vi "Robotiq Control.vi"() -> ()   [LabVIEW 2013]
uses:
  Common/controls/Robotiq Mode.ctl
  Common/classes/MF3/MF3.lvclass
  robotiq_labview/Class/Robotiq.lvclass
  Common/controls/Robotiq Positions.ctl
  labview_ros/std_msgs/Bool.ctl
  <vilib>/Platform/TimedLoop/XDataNode/timing_clust.ctl
  <vilib>/Platform/TimedLoop/XDataNode/nitl_modes.ctl
  <vilib>/Platform/TimedLoop/XDataNode/wakeup.ctl
  labview_ros/takktile_msgs/RobotiqTouch.ctl
  robotiq_labview/Controls/Gripper Command.ctl
  robotiq_labview/Controls/Finger Command.ctl
  <vilib>/Analysis/baseanly.llb/Unit Vector (DBL).vi
  <vilib>/Analysis/1siggen.llb/Riffle Array (I32) (obs 2012).vi
  <userlib>/_matio/level5/Public/Write/Append Data Element.llb/Append Data Element (1D Array of Double).vi
  <userlib>/_matio/level5/Public/Write/Append Data Element.llb/Append Data Element (2D Array of Double).vi
  <vilib>/Platform/TimedLoop/XDataNode/XDataNode.xnode
  <userlib>/_matio/level5.lvlib
  <vilib>/Platform/TimedLoop/XDataNode/XDNodeRunTimeDep.lvlib
  <vilib>/Analysis/NI_AALBase.lvlib
panel:
  in  "Gains":dbl[](array[numeric])=[3.0, 3.0, 3.0, 0.0, 0.0, 0.0, 0.0, 0.0, 0.0]
  out "Finger 3":T1
  out "Finger 2":T1
  out "Finger 1":T1
  out "Takktile Sender":errorcluster
  in  "Takktile":T2={"IP"="192.168.0.10", "Read Port"=5051, "Write Port"=5052}
  in  "Zero Takktile":bool
  out "Target Grasp":cluster{"Mode":T3, "Number":i32}={"Mode"=enum."Basic", "Number"=0}
  in  "OK Button":bool
  out "dp":T4(graph)
  out "velocities":T4(graph)
  out "area":dbl(graph)
  out "Requested?":bool caption="Time has Elapsed"
  in  "Transition time (s)":dbl=0.5 caption="Time Target (s)"
  out "Robotiq Mode":T3
  out "Takktile Rate":dbl
  in  "MasterFinger":T5={"PID Gains"={"Proportional Gain"=20, "Integral Gain"=5, "Derivative Gain"=0}, "Current limit"=0.0}
  in  "Data Logging":cluster{"Path":path, "Save":bool}={"Path"=path "c:/ni-rt/testing/grasping.mat", "Save"=TRUE}
  out "Logging Status":errorcluster
  out "Takktile Receiver":errorcluster
  in  "Robotiq Hand":cluster{"IP":string, "Port":u16, "Move":bool}={"IP"="192.168.0.8", "Port"=502, "Move"=FALSE}
  out "Robotiq Status":errorcluster
  out "MasterFinger Status":errorcluster
  in  "Stop":bool
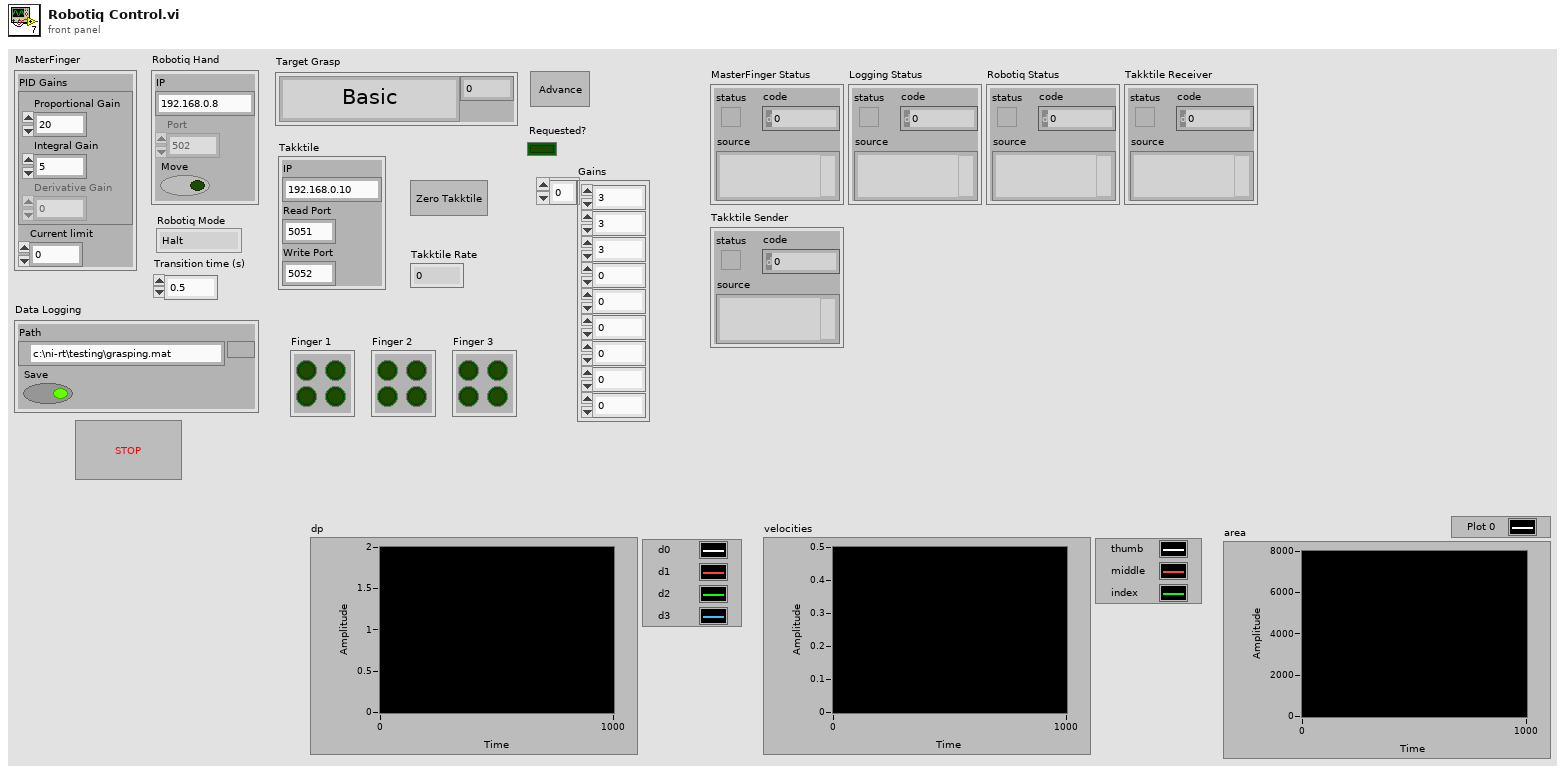
[diagram p1: front panel]
types:
  T1 = cluster{"tr":bool, "br":bool, "tl":bool, "bl":bool}
  T2 = cluster{"IP":string, "Read Port":u16, "Write Port":u16}
  T3 = typedef "Robotiq Mode.ctl" = enum16{"Halt", "Basic", "Scissor", "Ring", "Pinch"}
  T4 = cluster{"Vectors Norm[0]":dbl, "Vectors Norm[1]":dbl, "Vectors Norm[2]":dbl, "Vectors Norm[3]":dbl, "Vectors Norm[4]":dbl, "Vectors Norm[5]":dbl, "Vectors Norm[6]":dbl, "Vectors Norm[7]":dbl, "Vectors Norm[8]":dbl}
  T5 = cluster{"PID Gains":cluster{"Proportional Gain":i16, "Integral Gain":i16, "Derivative Gain":i16}, "Current limit":dbl}
  T6 = typedef "Robotiq Positions.ctl" = cluster{"Finger A":dbl, "Finger B":dbl, "Finger C":dbl, "Scissor":dbl}
  T7 = enum16{"big-endian, network order", "native, host order", "little-endian"}
  T8 = typedef "RobotiqTouch.ctl" = cluster{"f0":sgl[], "f1":sgl[], "f2":sgl[]}
  T9 = typedef "Bool.ctl" = cluster{"data":bool}
  T10 = typedef "XDNodeRunTimeDep.lvlib/timing_clust.ctl" = cluster{"Expected End [f-1]":u64, "Actual End [f-1]":u64, "Finished Late? [f-1]":bool, "Expected End [i-1]":u64, "Actual End [i-1]":u64, "Finished Late? [i-1]":bool, "Expected Start [i]":u64, "Actual Start [i]":u64, "Expected Start [f]":u64, "Actual Start [f]":u64, "Source Name":string, "Structure Name":string, "Period":i64, "Deadline":i64, "Offset":i64, "Start":i64, "Priority":i32, "Timeout":i32, "Mode":T11, "Wakeup Reason":T12, "Error":errorcluster, "Source Type":string, "Secondary Source Type":string, "Global End Time":u64, "Global Start Time":u64, "Frame Duration":u64, "Iteration Duration":u64, "Assigned CPU":i32, "I/O Scan Engine Mode":u32}
  T11 = typedef "XDNodeRunTimeDep.lvlib/nitl_modes.ctl" = enum32{"No Change", "Process missed periods, maintain original phase", "Discard missed periods, maintain original phase", "Process missed periods, ignore original phase", "Discard missed periods, ignore original phase"}
  T12 = typedef "XDNodeRunTimeDep.lvlib/wakeup.ctl" = enum32{"Normal", "Aborted", "Asynchronous wakeup", "Timing source error", "Timed loop error", "Timeout"}
  T13 = cluster{"Proportional Gain":i16, "Integral Gain":i16, "Derivative Gain":i16}
  T14 = typedef "Gripper Command.ctl" = cluster{"Finger A":T15, "Finger B":T15, "Finger C":T15, "Scissor":T15}
  T15 = typedef "Finger Command.ctl" = cluster{"Position":u8, "Speed":u8, "Force":u8}
  T16 = typedef "Gripper Status.ctl" = cluster{"Finger A":T17, "Finger B":T17, "Finger C":T17, "Scissor":T17, "Fault?":bool, "Activated?":bool}
  T17 = typedef "Finger Status.ctl" = cluster{"Position":dbl, "Current":dbl}
  T18 = typedef "Vector3D Fingers.ctl" = cluster{"Thumb":dbl[], "Middle":dbl[], "Index":dbl[]}
  T19 = cluster{"d":dbl[], "dp":dbl[], "dpp":dbl[], "area":dbl, "areap":dbl}
  T20 = cluster{"Velocities Norm 2[0]":dbl, "Velocities Norm 2[1]":dbl, "Velocities Norm 2[2]":dbl, "Velocities Norm 2[3]":dbl, "Velocities Norm 2[4]":dbl, "Velocities Norm 2[5]":dbl, "Velocities Norm 2[6]":dbl, "Velocities Norm 2[7]":dbl, "Velocities Norm 2[8]":dbl}
  T21 = cluster{"dp[0]":dbl, "dp[1]":dbl, "dp[2]":dbl, "dp[3]":dbl, "dp[4]":dbl, "dp[5]":dbl, "dp[6]":dbl, "dp[7]":dbl, "dp[8]":dbl}
  T22 = enum16{"open", "replace", "create", "open or create", "replace or create", "replace or create with confirmation"}
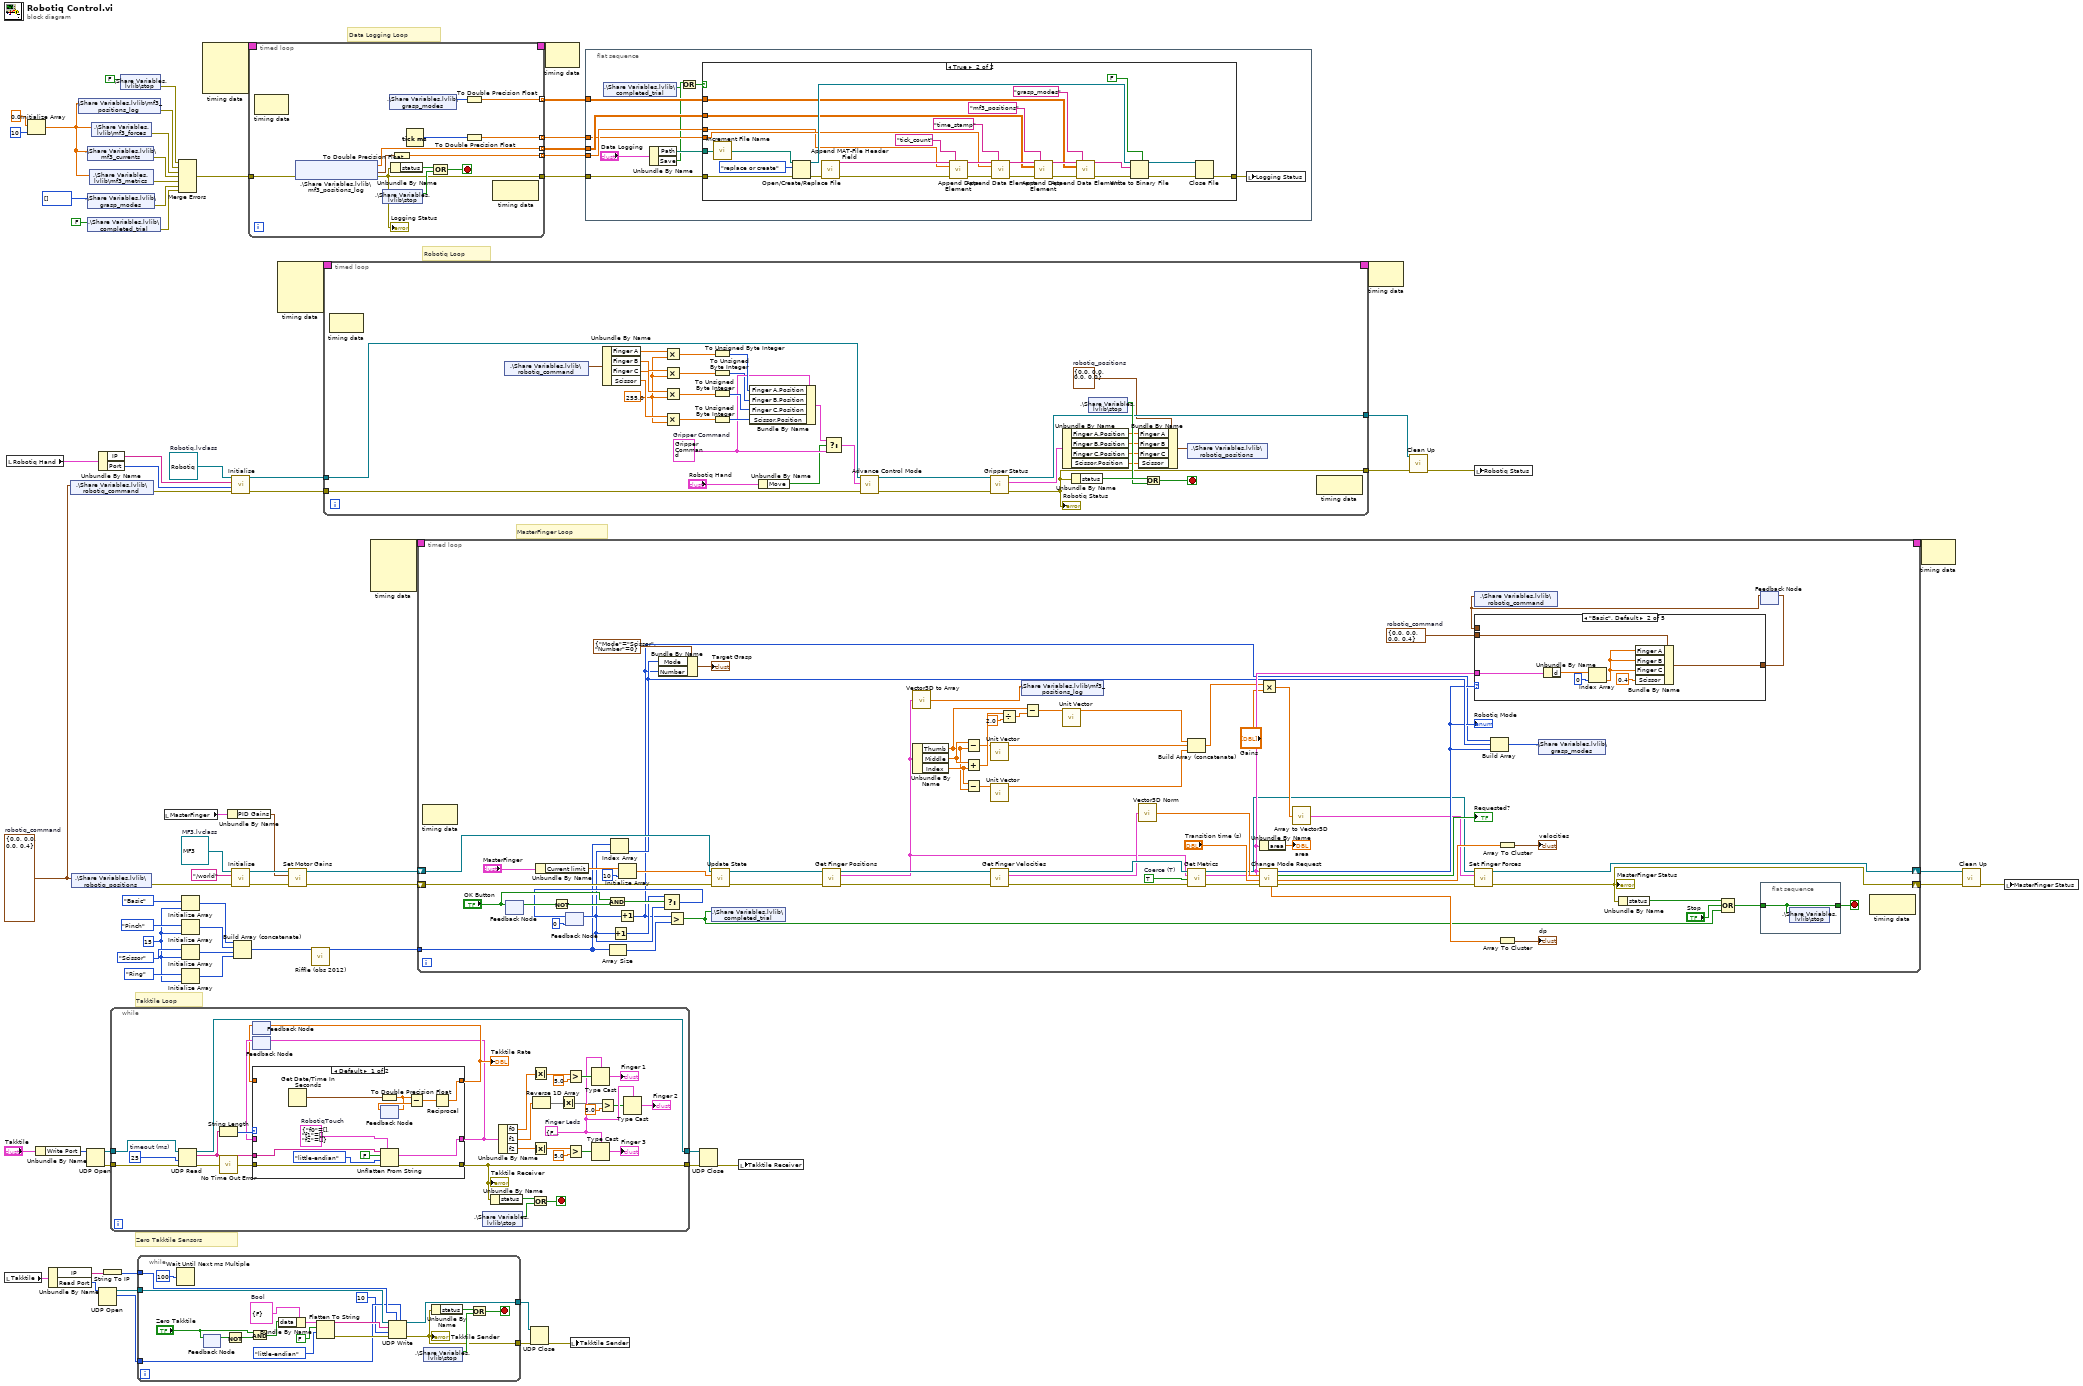
[diagram p0: block diagram]
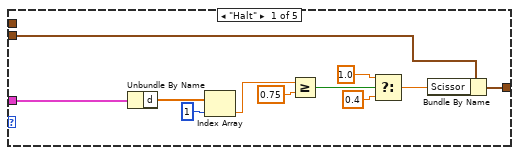
[diagram p3: hidden frame]
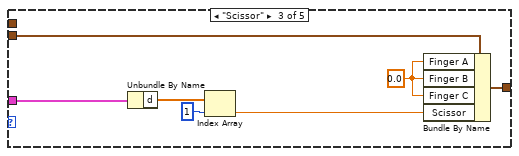
[diagram p4: hidden frame]
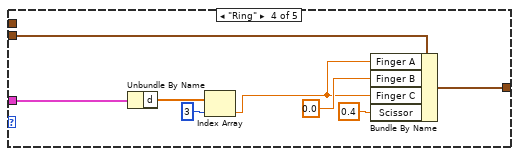
[diagram p5: hidden frame]
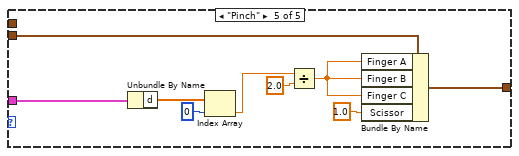
[diagram p6: hidden frame]
diagram:
  w20 = 15 ("dimension size")
  w36 = T6 {"Finger A"=0.0, "Finger B"=0.0, "Finger C"=0.0, "Scissor"=0.4}  # robotiq_command
  w72 = refnum<class "Robotiq.lvclass"> refnum  # Robotiq.lvclass
  w75 = refnum<class "MF3.lvclass"> refnum  # MF3.lvclass
  # "Zero Takktile Sensors"
  # "Data Logging Loop"
  # "Takktile Loop"
  # "Robotiq Loop"
  # "MasterFinger Loop"
  n1 = local read "Takktile"() -> (w9:T2)
  n2 = local read "Robotiq Hand"() -> (w29:cluster{"IP":string, "Port":u16, "Move":bool})
  n3 = Initialize Array "Initialize Array"(0.0 ("element"), 10 ("dimension size")) -> (w39:dbl[])
  n4 = Unbundle By Name("Takktile") -> ("Write Port"=w58:u16)
  n5 = Unbundle By Name(w9) -> ("IP"=w8:string, "Read Port"=w7:u16)
  n6 = shared-variable ".\\Share Variables.lvlib\\robotiq_command"(w36) -> (error out=w38:errorcluster)  [unwired: 1 in]
  n7 = shared-variable ".\\Share Variables.lvlib\\robotiq_positions"(w36) -> (error out=w37:errorcluster)  [unwired: 1 in]
  n8 = shared-variable ".\\Share Variables.lvlib\\mf3_positions_log"(w39) -> (error out=w63:errorcluster)  [unwired: 1 in]
  n9 = UDP Open(11:w58) -> (port=w57:refnum<k16>, 0:w56:errorcluster)  [unwired: 1 in, 4 out]
  n10 = shared-variable ".\\Share Variables.lvlib\\completed_trial"(FALSE ("completed_trial")) -> (error out=w12:errorcluster)  [unwired: 1 in]
  n11 = shared-variable ".\\Share Variables.lvlib\\mf3_currents"(w39) -> (error out=w61:errorcluster)  [unwired: 1 in]
  n12 = shared-variable ".\\Share Variables.lvlib\\grasp_modes"(i16[] [] ("grasp_modes")) -> (error out=w15:errorcluster)  [unwired: 1 in]
  n13 = shared-variable ".\\Share Variables.lvlib\\mf3_metrics"(w39) -> (error out=w40:errorcluster)  [unwired: 1 in]
  n14 = shared-variable ".\\Share Variables.lvlib\\mf3_forces"(w39) -> (error out=w62:errorcluster)  [unwired: 1 in]
  n15 = UDP Open(11:w7) -> (port=w6:refnum<k16>, 2:w4:u16)  [unwired: 1 in, 4 out]
  n16 = Unbundle By Name(w29) -> ("IP"=w67:string, "Port"=w66:u16)
  n17 = String To IP(1:w8) -> (0:w5:u32)
  n18 = while {
    tunnel: w57 -> [w103]
    tunnel: w56 -> [w102]
    tunnel: [w101] -> w55
    tunnel: [w98] -> w54
    stop <- w97 stop-if-true
    w86 = T1 {"tr"=FALSE, "br"=FALSE, "tl"=FALSE, "bl"=FALSE}  # Finger Leds
    w104 = 25  # timeout (ms)
    n19 = UDP Read(connection ID=w103, timeout ms (25000)=w104, 8:w102) -> (data out=w106:string, error out=w108:errorcluster, 3:w101:refnum<k16>)  [unwired: 1 in, 2 out]
    n20 = String Length(string=w106) -> (length=w107:i32)
    n21 = call <vilib>:"No Time Out Error.vi"("error in (no error)"=w108) -> ("error out"=w105:errorcluster)  [unwired: 14 out]
    n22 = feedback #1() -> (w95:dbl)  [unwired: 1 in]
    n23 = feedback #2() -> (w99:T8)  [unwired: 1 in]
    n24 = case shown="Default" w107 {
      tunnel: w106 -> [w119 _]
      tunnel: w105 -> [w118 w123]
      tunnel: [w117 w123] -> w98
      tunnel: [w113 w122] -> w93
      tunnel: w99 -> [_ w122]
      tunnel: [w114 w121] -> w96
      tunnel: w95 -> [_ w121]
      frame Default {
        w112 = T8 {"f0"=[], "f1"=[], "f2"=[]}  # RobotiqTouch
        n25 = Get Date/Time In Seconds() -> (seconds since 1Jan1904=w111:timestamp)
        n26 = To Double Precision Float(number=w111) -> (double precision float=w110:dbl)
        n27 = feedback #3() -> (w115:dbl)  [unwired: 1 in]
        n28 = feedback-in #3(w110) -> ()
        n29 = Unflatten From String(type=w112, binary string=w119, data includes array or string size? (T)=FALSE, byte order (0:big-endian, network order)=T7."little-endian", error in (no error)=w118) -> (value=w113:T8, error out=w117:errorcluster)  [unwired: 1 out]
        n30 = Subtract(x=w110, y=w115) -> (x-y=w109:dbl)
        n31 = Reciprocal(x=w109) -> (1/x=w114:dbl)
      }
      frame 0 {
      }
    }
    "Takktile Receiver" <- w98
    "Takktile Rate" <- w96
    n32 = feedback-in #1(w96) -> ()
    n33 = feedback-in #2(w93) -> ()
    n34 = shared-variable ".\\Share Variables.lvlib\\stop"() -> (w94:bool)  [unwired: 1 in, 1 out]
    n35 = Unbundle By Name(w98) -> ("status"=w100:bool)
    n36 = Unbundle By Name(w93) -> ("f0"=w90:sgl[], "f1"=w77:sgl[], "f2"=w78:sgl[])
    n37 = Or(x=w100, y=w94) -> (x .or. y?=w97:bool)
    n38 = Absolute Value(x=w90) -> (abs(x)=w91:sgl[])
    n39 = Absolute Value(x=w78) -> (abs(x)=w80:sgl[])
    n40 = Reverse 1D Array(array=w77) -> (reversed array=w76:sgl[])
    n41 = Absolute Value(x=w76) -> (abs(x)=w83:sgl[])
    n42 = Greater?(x=w91, y=sgl 5.0) -> (0:w89:bool[])
    n43 = Greater?(x=w80, y=sgl 5.0) -> (0:w79:bool[])
    n44 = Type Cast(type=w86, x=w89) -> (*(type *) &x=→"Finger 1":T1)
    n45 = Type Cast(type=w86, x=w79) -> (*(type *) &x=→"Finger 3":T1)
    n46 = Greater?(x=w83, y=sgl 5.0) -> (0:w82:bool[])
    n47 = Type Cast(type=w86, x=w82) -> (*(type *) &x=→"Finger 2":T1)
  }
  n48 = shared-variable ".\\Share Variables.lvlib\\stop"(FALSE ("stop")) -> (error out=w64:errorcluster)  [unwired: 1 in]
  n49 = while {
    tunnel: w6 -> [w134]
    tunnel: w5 -> [w133]
    tunnel: w4 -> [w132]
    tunnel: [w128] -> w3
    tunnel: [w127] -> w2
    stop <- w129 stop-if-true
    w138 = T9 {"data"=FALSE}  # Bool
    n50 = Wait Until Next ms Multiple(millisecond multiple=u32 100) -> ()  [unwired: 1 out]
    n51 = feedback #4() -> (w142:bool)  [unwired: 1 in]
    n52 = feedback-in #4("Zero Takktile") -> ()
    n53 = Not(x=w142) -> (.not. x?=w143:bool)
    n54 = And(x="Zero Takktile", y=w143) -> (x .and. y?=w124:bool)
    n55 = Bundle By Name(cluster=w138, "data"=w124) -> (w137:T9)
    n56 = Flatten To String(anything=w137, prepend array or string size? (T)=FALSE, byte order (0:big-endian, network order)=T7."little-endian") -> (data string=w136:string, error out=w135:errorcluster)  [unwired: 1 in, 1 out]
    n57 = UDP Write(address=w133, port or service name=w132, connection ID=w134, data in=w136, 8:w135, 9:10 ("timeout ms (25000)")) -> (error out=w127:errorcluster, 3:w128:refnum<k16>)
    "Takktile Sender" <- w127
    n58 = shared-variable ".\\Share Variables.lvlib\\stop"() -> (w130:bool)  [unwired: 1 in, 1 out]
    n59 = Unbundle By Name(w127) -> ("status"=w131:bool)
    n60 = Or(x=w131, y=w130) -> (x .or. y?=w129:bool)
  }
  n61 = local read "MasterFinger"() -> (w43:T5)
  n62 = Merge Errors(w64, w63, w62, w61, w40, w15, w12) -> (w47:errorcluster)
  n63 = Initialize Array(Robotiq_Mode."Basic" ("Robotiq Mode"), w20) -> (w26:T3[])
  n64 = Initialize Array(Robotiq_Mode."Pinch" ("Robotiq Mode"), w20) -> (w24:T3[])
  n65 = Initialize Array(Robotiq_Mode."Scissor" ("Robotiq Mode"), w20) -> (w22:T3[])
  n66 = Initialize Array(Robotiq_Mode."Ring" ("Robotiq Mode"), w20) -> (w19:T3[])
  n67 = node-c288() -> (w33:T10)  [unwired: 4 in]
  n68 = Unbundle By Name(w43) -> ("PID Gains"=w42:T13)
  n69 = call "Initialise.vi"("error in (no error)"=w38, "Port"=w66, "IP Address"=w67, "Robotiq in"=w72) -> ("error out"=w70:errorcluster, "Robotiq out"=w71:refnum<class "Robotiq.lvclass">)  [unwired: 6 in]
  n70 = call "Initialise.vi"("error in (no error)"=w37, "frame"="/world", "MF3 in"=w75) -> ("error out"=w44:errorcluster, "MF3 out"=w45:refnum<class "MF3.lvclass">)  [unwired: 7 in]
  n71 = Build Array (concatenate)(w26, w24, w22, w19) -> (w17:T3[])
  n72 = timed-loop {
    tunnel: [w151] -> w46
    tunnel: w47 -> [w155]
    tunnel: [w148] -> w50 mode=indexing
    tunnel: [w147] -> w49 mode=indexing
    tunnel: [w146] -> w48 mode=indexing
    timing: w33 -> [_]
    timing-out: [_] -> w32
    tunnel: [w144] -> w14 mode=indexing
    stop <- w152 stop-if-true
    n73 = node-c288() -> ()  [unwired: 1 in, 1 out]
    n74 = shared-variable ".\\Share Variables.lvlib\\mf3_positions_log"(error in=w155) -> (w148:dbl[], error out=w151:errorcluster, w149:timestamp)
    "Logging Status" <- w151
    n75 = shared-variable ".\\Share Variables.lvlib\\stop"() -> (w154:bool)  [unwired: 1 in, 1 out]
    n76 = shared-variable ".\\Share Variables.lvlib\\grasp_modes"() -> (w145:i16[])  [unwired: 1 in, 1 out]
    n77 = Unbundle By Name(w151) -> ("status"=w153:bool)
    n78 = To Double Precision Float(number=w149) -> (double precision float=w147:dbl)
    n79 = Tick Count (ms)() -> (millisecond timer value=w150:u32)
    n80 = Compound Arithmetic op=OR(w153, w154) -> (w152:bool)
    n81 = To Double Precision Float(number=w145) -> (double precision float=w144:dbl[])
    n82 = To Double Precision Float(number=w150) -> (double precision float=w146:dbl)
    n83 = node-c288() -> ()  [unwired: 1 in, 1 out]
  }
  n84 = node-c288() -> (w31:T10)  [unwired: 4 in]
  n85 = call "Set Motor Gains.vi"("error in (no error)"=w44, "motor gains"=w42, "MF3 in"=w45) -> ("error out"=w27:errorcluster, "MF3 out"=w28:refnum<class "MF3.lvclass">)  [unwired: 7 in]
  n86 = call-poly <vilib>:"Riffle (obs 2012).vi"("X"=w17) -> ("Riffled {X}"=w16:i32[])  [unwired: 8 in, 2 out]
  n87 = timed-loop {
    tunnel: w70 -> [w189]
    tunnel: [w179] -> w68
    tunnel: w71 -> [w190]
    tunnel: [w178] -> w69
    timing: w31 -> [_]
    timing-out: [_] -> w30
    stop <- w191 stop-if-true
    w175 = T6 {"Finger A"=0.0, "Finger B"=0.0, "Finger C"=0.0, "Scissor"=0.0}  # robotiq_positions
    w158 = 255.0 ("y")
    w167 = T14 {"Finger A"={"Position"=0, "Speed"=255, "Force"=255}, "Finger B"={"Position"=0, "Speed"=255, "Force"=255}, "Finger C"={"Position"=0, "Speed"=255, "Force"=255}, "Scissor"={"Position"=0, "Speed"=255, "Force"=255}}  # Gripper Command
    n88 = node-c288() -> ()  [unwired: 1 in, 1 out]
    n89 = shared-variable ".\\Share Variables.lvlib\\robotiq_command"() -> (w176:T6)  [unwired: 1 in, 1 out]
    n90 = Unbundle By Name(w176) -> ("Finger A"=w169:dbl, "Finger B"=w159:dbl, "Finger C"=w162:dbl, "Scissor"=w163:dbl)
    n91 = Multiply(x=w169, y=w158) -> (x*y=w187:dbl)
    n92 = Multiply(x=w159, y=w158) -> (x*y=w161:dbl)
    n93 = Multiply(x=w162, y=w158) -> (x*y=w185:dbl)
    n94 = Multiply(x=w163, y=w158) -> (x*y=w183:dbl)
    n95 = To Unsigned Byte Integer(number=w187) -> (unsigned 8bit integer=w186:u8)
    n96 = To Unsigned Byte Integer(number=w161) -> (unsigned 8bit integer=w160:u8)
    n97 = To Unsigned Byte Integer(number=w185) -> (unsigned 8bit integer=w184:u8)
    n98 = To Unsigned Byte Integer(number=w183) -> (unsigned 8bit integer=w182:u8)
    n99 = Bundle By Name(cluster=w167, "Finger A.Position"=w186, "Finger B.Position"=w160, "Finger C.Position"=w184, "Scissor.Position"=w182) -> (w168:T14)
    n100 = Unbundle By Name("Robotiq Hand") -> ("Move"=w164:bool)
    n101 = Select(t=w168, s=w164, f=w167) -> (s? t:f=w166:T14)
    n102 = call "Advance Control Mode.vi"("error in (no error)"=w189, "Gripper Command"=w166, "Robotiq in"=w190) -> ("error out"=w180:errorcluster, "Robotiq out"=w181:refnum<class "Robotiq.lvclass">)  [unwired: 7 in]
    n103 = call "Gripper Status.vi"("error in (no error)"=w180, "Robotiq in"=w181) -> ("error out"=w179:errorcluster, "Gripper Status"=w177:T16, "Robotiq out"=w178:refnum<class "Robotiq.lvclass">)  [unwired: 7 in]
    "Robotiq Status" <- w179
    n104 = Unbundle By Name(w177) -> ("Finger A.Position"=w174:dbl, "Finger B.Position"=w173:dbl, "Finger C.Position"=w172:dbl, "Scissor.Position"=w171:dbl)
    n105 = Unbundle By Name(w179) -> ("status"=w192:bool)
    n106 = shared-variable ".\\Share Variables.lvlib\\stop"() -> (w188:bool)  [unwired: 1 in, 1 out]
    n107 = Bundle By Name(cluster=w175, "Finger A"=w174, "Finger B"=w173, "Finger C"=w172, "Scissor"=w171) -> (w170:T6)
    n108 = Or(x=w192, y=w188) -> (x .or. y?=w191:bool)
    n109 = shared-variable ".\\Share Variables.lvlib\\robotiq_positions"(w170) -> ()  [unwired: 1 in, 1 out]
    n110 = node-c288() -> ()  [unwired: 1 in, 1 out]
  }
  n111 = node-c288() -> (w35:T10)  [unwired: 4 in]
  n112 = timed-loop {
    shift-right: [w195] -> w73
    shift-left: w28 -> [w245]
    shift-right: [w197] -> w59
    shift-left: w27 -> [w244]
    timing: w35 -> [_]
    timing-out: [_] -> w34
    tunnel: w16 -> [w226]
    stop <- w218 stop-if-true
    w256 = T6 {"Finger A"=0.0, "Finger B"=0.0, "Finger C"=0.0, "Scissor"=0.4}  # robotiq_command
    w258 = TRUE  # Coerce (T)
    n113 = node-c288() -> ()  [unwired: 1 in, 1 out]
    n114 = feedback #5() -> (w234:bool)  [unwired: 1 in]
    n115 = feedback-in #5("OK Button") -> ()
    n116 = Unbundle By Name("MasterFinger") -> ("Current limit"=w262:dbl)
    n117 = Not(x=w234) -> (.not. x?=w233:bool)
    n118 = feedback #6(0 ("index")) -> (w229:i32)
    n119 = And(x="OK Button", y=w233) -> (x .and. y?=w232:bool)
    n120 = Array Size(array=w226) -> (size(s)=w225:i32)
    n121 = Index Array(array=w226, index=w229) -> (element=w224:i32)
    n122 = Increment(x=w229) -> (x+1=w230:i32)
    n123 = Increment(x=w229) -> (x+1=w220:i32)
    n124 = Initialize Array(w262, 10 ("dimension size")) -> (w260:dbl[])
    n125 = Bundle By Name(cluster=cluster{"Mode":T3, "Number":i32} {"Mode"=enum."Scissor", "Number"=0} ("Target Grasp"), "Mode"=w224, "Number"=w220) -> (→"Target Grasp":cluster{"Mode":T3, "Number":i32})
    n126 = Select(t=w230, s=w232, f=w229) -> (s? t:f=w231:i32)
    n127 = feedback-in #6(w231) -> ()
    n128 = Greater?(x=w220, y=w225) -> (0:w221:bool)
    n129 = call "Update State.vi"("error in (no error)"=w244, "current_limits"=w260, "MF3 in"=w245) -> ("error out"=w217:errorcluster, "MF3 out"=w216:refnum<class "MF3.lvclass">)  [unwired: 7 in]
    n130 = shared-variable ".\\Share Variables.lvlib\\completed_trial"(w221) -> ()  [unwired: 1 in, 1 out]
    n131 = call "Get Finger Positions.vi"("error in (no error)"=w217, "MF3 in"=w216) -> ("error out"=w251:errorcluster, "Finger Positions"=w211:T18, "MF3 out"=w254:refnum<class "MF3.lvclass">)  [unwired: 6 in, 1 out]
    n132 = call "Vector3D to Array.vi"("Vector3D"=w211) -> ("Array"=w264:dbl[])
    n133 = Unbundle By Name(w211) -> ("Thumb"=w207:dbl[], "Middle"=w210:dbl[], "Index"=w208:dbl[])
    n134 = Subtract(x=w210, y=w207) -> (x-y=w209:dbl[])
    n135 = Add(x=w210, y=w208) -> (x+y=w215:dbl[])
    n136 = Subtract(x=w208, y=w207) -> (x-y=w206:dbl[])
    n137 = call-poly <vilib>:"Unit Vector.vi"("Input Vector"=w209) -> ("Unit Vector"=w204:dbl[])  [unwired: 8 in, 2 out]
    n138 = call-poly <vilib>:"Unit Vector.vi"("Input Vector"=w206) -> ("Unit Vector"=w203:dbl[])  [unwired: 8 in, 2 out]
    n139 = call "Get Finger Velocities.vi"("error in (no error)"=w251, "MF3 in"=w254) -> ("error out"=w252:errorcluster, "Fingers Velocities"=w249:T18, "MF3 out"=w253:refnum<class "MF3.lvclass">)  [unwired: 6 in, 1 out]
    n140 = Divide(x=w215, y=2.0) -> (x/y=w213:dbl[])
    n141 = shared-variable ".\\Share Variables.lvlib\\mf3_positions_log"(w264) -> ()  [unwired: 1 in, 1 out]
    n142 = Subtract(x=w207, y=w213) -> (x-y=w212:dbl[])
    n143 = call-poly <vilib>:"Unit Vector.vi"("Input Vector"=w212) -> ("Unit Vector"=w205:dbl[])  [unwired: 8 in, 2 out]
    n144 = call "Vector3D Norm.vi"("Vector3D"=w249) -> ("Vectors Norm"=w242:dbl[])
    n145 = Build Array (concatenate)(w205, w204, w203) -> (w201:dbl[])
    n146 = call "Get Metrics.vi"("error in (no error)"=w252, "Coerce (T)"=w258, "Finger Positions"=w211, "MF3 in"=w253) -> ("error out"=w255:errorcluster, "metrics"=w238:T19, "MF3 out"=w196:refnum<class "MF3.lvclass">)  [unwired: 5 in]
    n147 = Unbundle By Name(w238) -> ("area"=→"area":dbl)
    n148 = call "Change Mode Request.vi"("error in (no error)"=w255, "Transition time (s)"="Transition time (s)", "Velocities Norm"=w242, "metrics"=w238) -> ("error out"=w198:errorcluster, "Velocities Norm 2"=w240:dbl[], "Requested?"=→"Requested?":bool, "Robotiq Mode"=w223:T3, "dp"=w237:dbl[])  [unwired: 3 in]
    "Robotiq Mode" <- w223
    n149 = Multiply(x=w201, y="Gains") -> (x*y=w199:dbl[])
    n150 = call "Array to Vector3D.vi"("Array"=w199) -> ("Vector3D"=w202:T18)
    n151 = call "Set Finger Forces.vi"("error in (no error)"=w198, "Finger Forces"=w202, "MF3 in"=w196) -> ("error out"=w197:errorcluster, "MF3 out"=w195:refnum<class "MF3.lvclass">)  [unwired: 6 in, 1 out]
    "MasterFinger Status" <- w197
    n152 = Build Array(w220, w224, w223) -> (w222:i32[])
    n153 = Array To Cluster(array=w240) -> (cluster=→"velocities":T20)
    n154 = Array To Cluster(array=w237) -> (cluster=→"dp":T21)
    n155 = shared-variable ".\\Share Variables.lvlib\\grasp_modes"(w222) -> ()  [unwired: 1 in, 1 out]
    n156 = Unbundle By Name(w197) -> ("status"=w257:bool)
    n157 = Compound Arithmetic op=OR(w257, "Stop", w221) -> (w219:bool)
    n158 = feedback #7() -> (w246:T6)  [unwired: 1 in]
    n159 = shared-variable ".\\Share Variables.lvlib\\robotiq_command"(w246) -> ()  [unwired: 1 in, 1 out]
    n160 = case shown="\"Basic\", Default" w223 {
      tunnel: w238 -> [w273 w285 w290 w298 w308]
      tunnel: w256 -> [w268 w283 w289 w299 w307]
      tunnel: [w278 w280 w288 w295 w306] -> w247
      tunnel: w246 -> [_ _ _ _ _]
      frame "Halt" {
        n161 = Unbundle By Name(w273) -> ("d"=w274:dbl[])
        n162 = Index Array(array=w274, index=1) -> (element=w275:dbl)
        n163 = Greater Or Equal?(x=w275, y=0.75) -> (x >= y?=w272:bool)
        n164 = Select(t=1.0 ("Scissor"), s=w272, f=0.4 ("Scissor")) -> (s? t:f=w269:dbl)
        n165 = Bundle By Name(cluster=w268, "Scissor"=w269) -> (w278:T6)
      }
      frame "Basic", Default {
        n166 = Unbundle By Name(w285) -> ("d"=w284:dbl[])
        n167 = Index Array(array=w284, index=0) -> (element=w282:dbl)
        n168 = Bundle By Name(cluster=w283, "Finger A"=w282, "Finger B"=w282, "Finger C"=w282, "Scissor"=0.4) -> (w280:T6)
      }
      frame "Scissor" {
        w286 = 0.0 ("Finger C")
        n169 = Unbundle By Name(w290) -> ("d"=w292:dbl[])
        n170 = Index Array(array=w292, index=1) -> (element=w287:dbl)
        n171 = Bundle By Name(cluster=w289, "Finger A"=w286, "Finger B"=w286, "Finger C"=w286, "Scissor"=w287) -> (w288:T6)
      }
      frame "Ring" {
        n172 = Unbundle By Name(w298) -> ("d"=w296:dbl[])
        n173 = Index Array(array=w296, index=3) -> (element=w293:dbl)
        n174 = Bundle By Name(cluster=w299, "Finger A"=w293, "Finger B"=0.0 ("Finger C"), "Finger C"=w293, "Scissor"=0.4) -> (w295:T6)
      }
      frame "Pinch" {
        n175 = Unbundle By Name(w308) -> ("d"=w305:dbl[])
        n176 = Index Array(array=w305, index=0) -> (element=w302:dbl)
        n177 = Divide(x=w302, y=2.0) -> (x/y=w301:dbl)
        n178 = Bundle By Name(cluster=w307, "Finger A"=w301, "Finger B"=w301, "Finger C"=w301, "Scissor"=1.0) -> (w306:T6)
      }
    }
    n179 = feedback-in #7(w247) -> ()
    n180 = flat-sequence {
      tunnel: w219 -> [w265]
      tunnel: [w265] -> w218
      frame #0 {
        n181 = shared-variable ".\\Share Variables.lvlib\\stop"(w265) -> ()  [unwired: 1 in, 1 out]
      }
    }
    n182 = node-c288() -> ()  [unwired: 1 in, 1 out]
  }
  n183 = UDP Close(connection ID=w3, 8:w2) -> (error out=w1:errorcluster)  [unwired: 1 out]
  n184 = node-c288(w32) -> ()  [unwired: 1 out]
  n185 = local write "Takktile Sender"(w1) -> ()
  n186 = flat-sequence {
    tunnel: w50 -> [w319]
    tunnel: w49 -> [w318]
    tunnel: w48 -> [w317]
    tunnel: w46 -> [w316]
    tunnel: w14 -> [w313]
    frame #0 {
      n187 = shared-variable ".\\Share Variables.lvlib\\completed_trial"() -> (w310:bool)  [unwired: 1 in, 1 out]
      n188 = Unbundle By Name("Data Logging") -> ("Path"=w314:path, "Save"=w312:bool)
      n189 = Or(x=w312, y=w310) -> (x .or. y?=w311:bool)
      n190 = case shown="True" w311 {
        tunnel: [w321 w334] -> w320
        tunnel: w319 -> [_ w333]
        tunnel: w318 -> [_ w332]
        tunnel: w317 -> [_ w331]
        tunnel: w316 -> [w321 w330]
        tunnel: w314 -> [_ w328]
        tunnel: w313 -> [_ w322]
        frame False {
        }
        frame True {
          n191 = call "Increment File Name.vi"("Full Path"=w328) -> ("New Path"=w335:path)
          n192 = Open/Create/Replace File(file path (use dialog)=w335, error in=w330, operation (0:open)=T22."replace or create") -> (refnum out=w336:refnum<file>, error out=w329:errorcluster)  [unwired: 3 in, 1 out]
          n193 = call <userlib>:"Append MAT-File Header Field.vi"("error"=w329) -> ("result string"=w345:string, "error out"=w344:errorcluster)  [unwired: 13 in]
          n194 = call-poly <userlib>:"Append Data Element.vi"("initial string"=w345, "Data Name"="tick_count", "data"=w331, "error in"=w344) -> ("result string"=w339:string, "error out"=w338:errorcluster)  [unwired: 10 in]
          n195 = call-poly <userlib>:"Append Data Element.vi"("initial string"=w339, "Data Name"="time_stamp", "data"=w332, "error in"=w338) -> ("result string"=w341:string, "error out"=w340:errorcluster)  [unwired: 10 in]
          n196 = call-poly <userlib>:"Append Data Element.vi"("initial string"=w341, "Data Name"="mf3_positions" ("array name"), "data"=w333, "error in"=w340) -> ("result string"=w327:string, "error out"=w326:errorcluster)  [unwired: 10 in]
          n197 = call-poly <userlib>:"Append Data Element.vi"("initial string"=w327, "Data Name"="grasp_modes" ("array name"), "data"=w322, "error in"=w326) -> ("result string"=w324:string, "error out"=w325:errorcluster)  [unwired: 10 in]
          n198 = Write to Binary File(file (use dialog)=w336, data=w324, error in=w325, 5:FALSE ("prepend array or string size? (T)")) -> (refnum out=w347:refnum<file>, error out=w346:errorcluster)  [unwired: 2 in, 1 out]
          n199 = Close File(refnum=w347, error in=w346) -> (error out=w334:errorcluster)  [unwired: 1 out]
        }
      }
      n200 = local write "Logging Status"(w320) -> ()
    }
  }
  n201 = UDP Close(connection ID=w55, 8:w54) -> (error out=w51:errorcluster)  [unwired: 1 out]
  n202 = local write "Takktile Receiver"(w51) -> ()
  n203 = node-c288(w30) -> ()  [unwired: 1 out]
  n204 = call "Clean Up.vi"("error in (no error)"=w68, "Robotiq in"=w69) -> ("error out"=w60:errorcluster)  [unwired: 8 in, 1 out]
  n205 = local write "Robotiq Status"(w60) -> ()
  n206 = node-c288(w34) -> ()  [unwired: 1 out]
  n207 = call "Clean Up.vi"("error in (no error)"=w59, "MF3 in"=w73) -> ("error out"=w41:errorcluster)  [unwired: 8 in, 1 out]
  n208 = local write "MasterFinger Status"(w41) -> ()
